vi "全局 1.vi"() -> ()   [LabVIEW 2022 SP3]
panel:
  out "是否正常平衡":bool
  out "是否匀速转动":bool
  out "是否起摆":bool
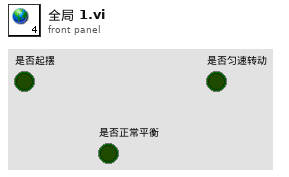
[diagram p1: front panel]
diagram:
